vi "Save VI by path.vi"(8 "error in (no error)":errorcluster, 11 "VI path":path) -> (0 "error out":errorcluster)   [LabVIEW 2016, in "NIVS_Consolidated_CDW_MetaDataObj.lvclass"]
doc: "Save the VI which the path input specifies."
uses:
  NIVS_Consolidated_CDW_MetaDataObj.lvclass
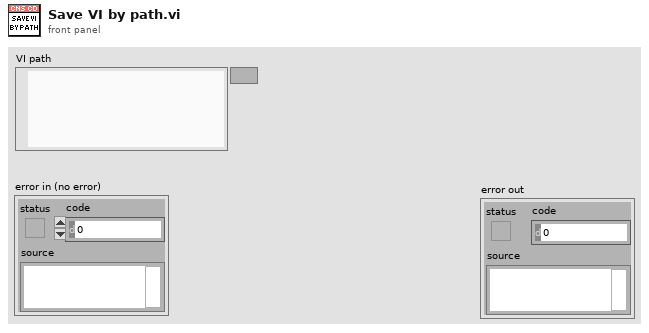
[diagram p1: front panel]
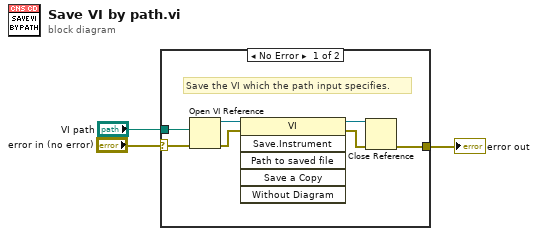
[diagram p0: block diagram]
diagram:
  n1 = case shown="No Error" "error in (no error)" {
    selector: "error in (no error)" -> [w5 w11]
    tunnel: "VI path" -> [w6 _]
    tunnel: [w4 w11] -> w2
    frame No Error {
      # "Save the VI which the path input specifies."
      n2 = Open VI Reference(vi path=w6, error in (no error)=w5) -> (vi reference=w10:refnum<vi>, error out=w9:errorcluster)  [unwired: 4 in]
      n3 = invoke class="VI" method="Save.Instrument"(reference=w10, error in=w9) -> (reference out=w8:refnum<vi>, error out=w7:errorcluster)  [unwired: 4 in, 4 out]
      n4 = Close Reference(reference=w8, error in (no error)=w7) -> (error out=w4:errorcluster)
    }
    frame Error {
      # "Output default values."
    }
  }
  "error out" <- w2
